vi "Add Line.vi"(8 "error in (no error)":errorcluster, 10 "Line":T1, 11 "GPIC ScaleAndLimit configuration in":refnum<class "GPIC ScaleAndLimit configuration.lvclass">) -> (0 "error out":errorcluster, 3 "GPIC ScaleAndLimit configuration out":refnum<class "GPIC ScaleAndLimit configuration.lvclass">)   [LabVIEW 2015, in "GPIC ScaleAndLimit configuration.lvclass"]
uses:
  GPIC ScaleAndLimit configuration.lvclass
  <vilib>/NI/Tag Bus Module Framework/channel/TBM channel.lvclass
  GPIC ScaleAndLimit configuration.lvclass/GPIC ScaleAndLimit configuration.ctl
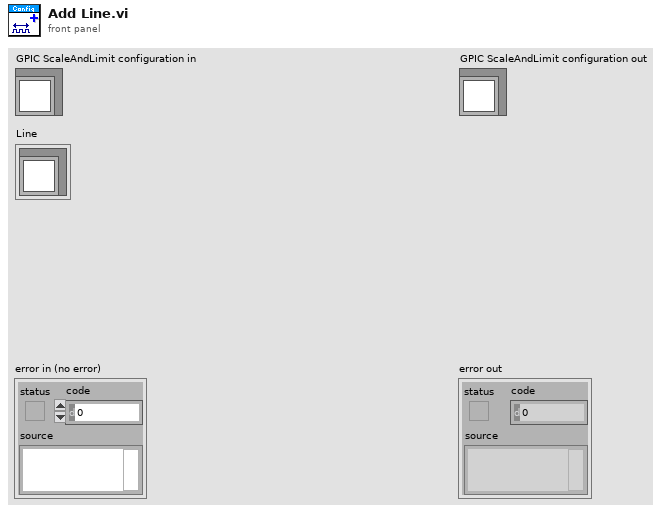
[diagram p1: front panel]
types:
  T1 = cluster{"channel":refnum<class "TBM channel.lvclass">}
  T2 = cluster{"channel":refnum<class "TBM channel.lvclass">}[]
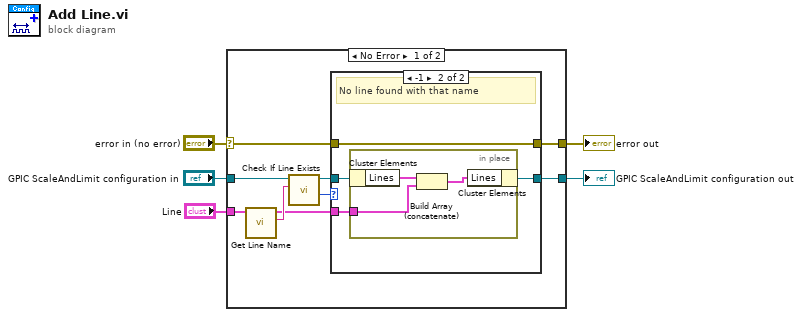
[diagram p0: block diagram]
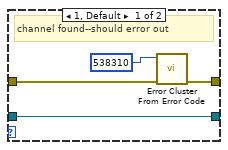
[diagram p2: hidden frame]
diagram:
  n1 = case shown="No Error" "error in (no error)" {
    selector: "error in (no error)" -> [w8 w27]
    tunnel: [w7 w27] -> w4
    tunnel: [w6 w26] -> w2
    tunnel: "GPIC ScaleAndLimit configuration in" -> [w12 w26]
    tunnel: "Line" -> [w14 _]
    frame No Error {
      n2 = call "Get Line Name.vi"("Line in"=w14) -> ("Name"=w13:string, "Line out"=w10:T1)  [unwired: 8 in, 1 out]
      n3 = call-dynamic "Check If Line Exists.vi"("name to locate"=w13, "GPIC ScaleAndLimit configuration in"=w12) -> ("index"=w9:i32, "GPIC ScaleAndLimit configuration out"=w11:refnum<class "GPIC ScaleAndLimit configuration.lvclass">)  [unwired: 5 in, 3 out]
      n4 = case shown="-1" w9 {
        tunnel: [w18 w21] -> w7
        tunnel: w8 -> [w16 w21]
        tunnel: w11 -> [w15 w20]
        tunnel: w10 -> [_ w22]
        tunnel: [w15 w19] -> w6
        frame 1, Default {
          # "channel found--should error out"
          n5 = call <vilib>:"Error Cluster From Error Code.vi"("error in (no error)"=w16, "error code (0)"=538310) -> ("error out"=w18:errorcluster)  [unwired: 7 in]
        }
        frame -1 {
          # "No line found with that name"
          n6 = in-place {
            in-place-border: w22 -> [w23]
            n7 = in-place-cluster #1(w20) -> ("Lines"=w24:T2)
            n8 = Build Array (concatenate)(w24, w23) -> (w25:T2)
            n9 = in-place-cluster #1("Lines"=w25) -> (w19:refnum<class "GPIC ScaleAndLimit configuration.lvclass">)
          }
        }
      }
    }
    frame Error {
    }
  }
  "error out" <- w4
  "GPIC ScaleAndLimit configuration out" <- w2
